vi "AppendStrArrayH5.vi"(6 "type name (default)":string, 8 "error in (no error)":errorcluster, 9 "Data":string[](array[string]), 10 "Data Dimension (array)":i32[](array[numeric]), 11 "dset in":T1 format="%.0x") -> (0 "error out":errorcluster)   [LabVIEW 2014]
uses:
  <vilib>/addons/h5labview2/base/hid_t.ctl
  <vilib>/addons/h5labview2/base/lib_path.vi
  <vilib>/addons/h5labview2/base/H5Equery.vi
  <vilib>/addons/h5labview2/dataset/H5Dwrite.llb/H5Dwrite.xnode
  <vilib>/addons/h5labview2/dataset/H5D.lvlib
  <vilib>/addons/h5labview2/space/H5S.lvlib
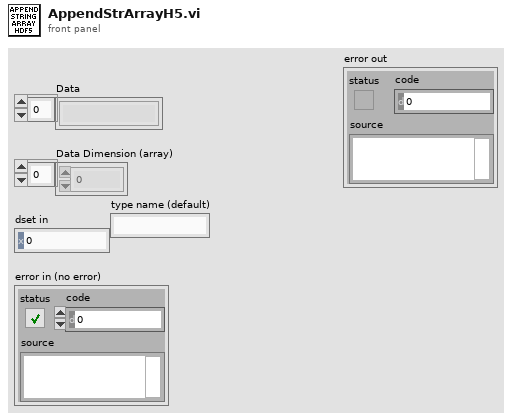
[diagram p1: front panel]
types:
  T1 = typedef "hid_t.ctl" = i32
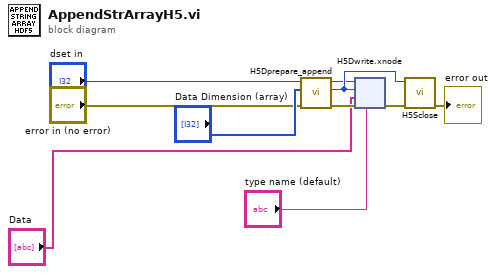
[diagram p0: block diagram]
diagram:
  n1 = call <vilib>:"H5Dprepare_append.vi"("error in (no error)"="error in (no error)", "append dims"="Data Dimension (array)", "dset in"="dset in") -> ("error out"=w6:errorcluster, "space out"=w8:T1, "dset out"=w7:T1)  [unwired: 6 in]
  n2 = xnode "H5Dwrite.xnode"("type name (default)"="type name (default)", "error in (no error)"=w6, "data"="Data", "file space"=w8, "ref in"=w7) -> ("error out"=w9:errorcluster)  [unwired: 2 in, 2 out]
  n3 = call <vilib>:"H5Sclose.vi"("error in (no error)"=w9, "space in"=w8) -> ("error out"=→"error out":errorcluster)  [unwired: 9 in]
